vi "get default error list.vi"(8 "error in (no error)":errorcluster, 11 "RT Resource Usage configuration in":refnum<class "RT Resource Usage configuration.lvclass">) -> (0 "error out":errorcluster, 2 "error list":T1[](array[typedef]), 3 "RT Resource Usage configuration out":refnum<class "RT Resource Usage configuration.lvclass">)   [LabVIEW 2017, in "RT Resource Usage configuration.lvclass"]
uses:
  RT Resource Usage configuration.lvclass
  <vilib>/NI/DCAF/Tag Editor Core/control module/configuration/error classification setting.ctl
  <vilib>/NI/Tag Bus Module Framework/runtime/error classification.ctl
  <vilib>/NI/Tag Bus Module Framework/runtime/TBM module execution interface.lvclass
  <vilib>/NI/DCAF/Tag Editor Core/control module/configuration/control module configuration.lvclass
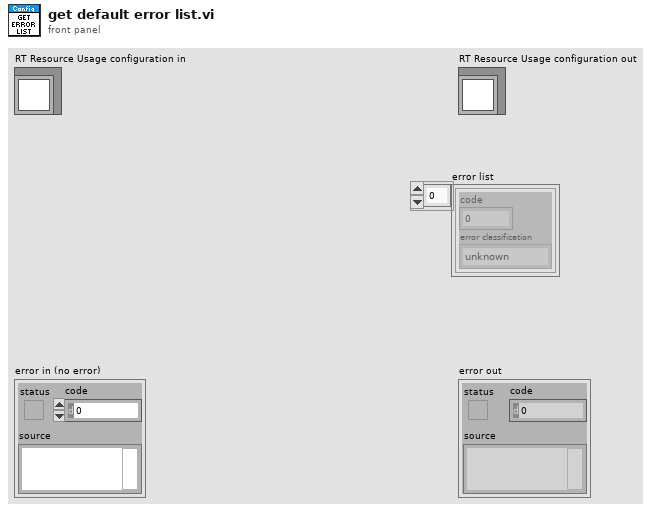
[diagram p1: front panel]
types:
  T1 = typedef "control module configuration.lvclass/error classification setting.ctl" = cluster{"code":i32, "error classification":T2}
  T2 = typedef "TBM module execution interface.lvclass/error classification.ctl" = enum16{"unknown", "none", "trivial", "recoverable", "critical"}
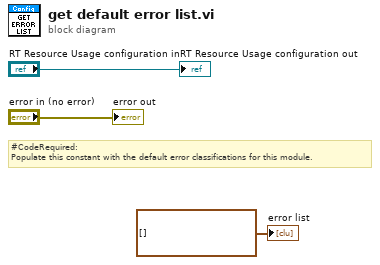
[diagram p0: block diagram]
diagram:
  # "#CodeRequired:\nPopulate this constant with the default error classifications for this module."
  "error out" <- "error in (no error)"
  "RT Resource Usage configuration out" <- "RT Resource Usage configuration in"
  "error list" <- T1[] [] ("error list")
